vi "Test Worker Waiting After Completing Job.vi"(8 "error in (no error)":errorcluster, 11 "Barista Test in":refnum<class "Barista Test.lvclass">) -> (0 "error out":errorcluster, 3 "Barista Test out":refnum<class "Barista Test.lvclass">)   [LabVIEW 2020, in "Barista Test.lvclass"]
uses:
  Barista Test.lvclass
  C:/Users/anton/Documents/GitHub/Triarc-Examples/Coffee Shop/Worker Test/Worker Test.lvclass
  C:/Program Files (x86)/National Instruments/LabVIEW 2020/vi.lib/Asteme/LUnit/Test Case.lvclass
  Stub Job Processor/Stub Job Handler.lvclass
  C:/Users/anton/Documents/GitHub/Triarc-Examples/Coffee Shop/Process Job/Job Handler.lvclass
  Stub Pick Up Order/Stub Pick Up Order.lvclass
  C:/Users/anton/Documents/GitHub/Triarc-Examples/Coffee Shop/Pick Up Order/Pick Up Order.lvclass
  Support/Beverages/Beverage/Beverage.lvclass
  <vilib>/Asteme/Triarc Framework/Process/Process.lvclass/Process.ctl
  <vilib>/Asteme/LUnit/Test Case.lvclass/Test Case.ctl
  <vilib>/Asteme/LUnit/LUnit Assertion Result.lvclass/LUnit Assertion Result.ctl
  <vilib>/Asteme/Triarc Framework Test Suite/Support/Execution timer.vi
  <vilib>/Asteme/Triarc Framework/Process/Private/SubVIs/Wait for finish.vi
  <vilib>/Asteme/Triarc Framework/Process/Protected/Messaging/Enqueue Message.vi
  <vilib>/Asteme/Triarc Framework/Process/Private/SubVIs/Set Lifecycle State.vi
  <vilib>/Asteme/Triarc Framework/Process/Public/Lifecycle/Get Lifecycle State.vi
  <vilib>/Asteme/LUnit/Palette/Pass If.vi
  <vilib>/Asteme/LUnit/Set Assertion Type.vi
  <vilib>/AdvancedString/1D String Array to Delimited String.vi
  <vilib>/Utility/error.llb/Clear Errors.vi
  <vilib>/Asteme/LUnit/Palette/Fail.vi
  <vilib>/Asteme/LUnit/Palette/Pass.vi
  <vilib>/Asteme/LUnit/LUnit Write Assertion Type.vi
  <vilib>/Asteme/LUnit/Add test result.vi
  <vilib>/Asteme/LUnit/LUnit Write Passed.vi
  <vilib>/Asteme/LUnit/LUnit Get Test Case.vi
  <vilib>/Asteme/LUnit/Assertion Result/LUnit Get Test Name.vi
  <vilib>/Asteme/LUnit/LUnit Write Message.vi
  <vilib>/Asteme/LUnit/LUnit Write Description.vi
  <vilib>/Asteme/LUnit/Read Test Case Name.vi
  Worker/Worker.lvclass
  C:/Program Files (x86)/National Instruments/LabVIEW 2020/vi.lib/Asteme/Triarc Framework/Process/Process.lvclass
  <vilib>/Asteme/Triarc Framework Test Suite/Support/Event Helpers/Dequeue Event Message.vi
  <vilib>/Utility/error.llb/Error Cluster From Error Code.vi
  <vilib>/Asteme/LUnit/LUnit Assertion Result.lvclass
  <vilib>/Asteme/Triarc Framework/Process/Process.lvclass
  Worker Test/Worker Test.lvclass
  <vilib>/Asteme/Triarc Framework Test Suite/Support/Event Helpers/Event Helpers.lvlib
  <vilib>/Asteme/LUnit/Test Case.lvclass
  Support/Order Item/Order Item.lvclass
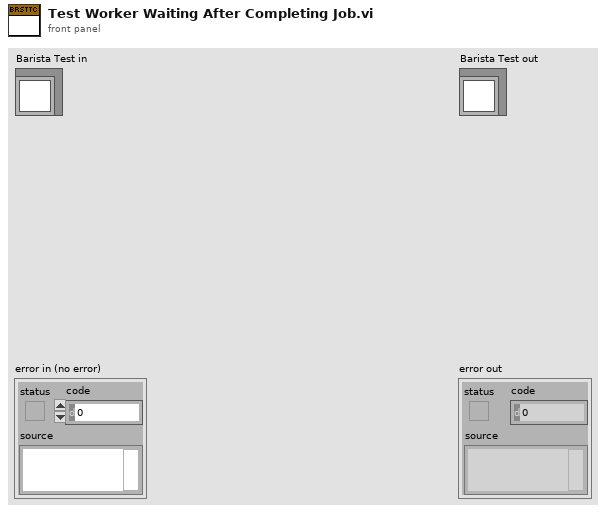
[diagram p1: front panel]
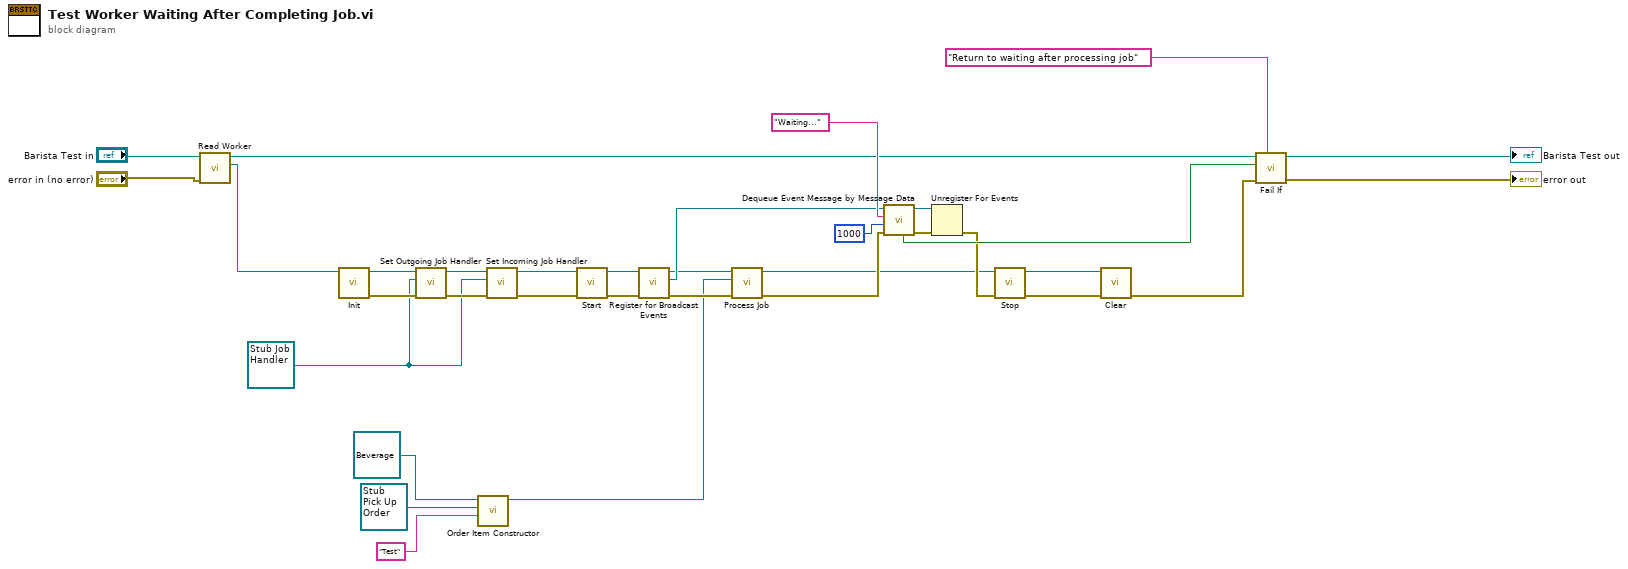
[diagram p0: block diagram]
diagram:
  w1 = refnum<class "Stub Job Handler.lvclass"> refnum ("Stub Job Processor.lvclass")
  n1 = call "Read Worker.vi"("error in (no error)"="error in (no error)", "Worker Test in"="Barista Test in") -> ("Worker"=w7:refnum<class "Worker.lvclass">, "Worker Test out"=w6:refnum<class "Barista Test.lvclass">)  [unwired: 7 in, 1 out]
  n2 = call-dynamic "Init.vi"("View In"=w7) -> ("error out"=w26:errorcluster, "View Out"=w25:refnum<class "Worker.lvclass">)  [unwired: 9 in]
  n3 = call "Set Outgoing Job Handler.vi"("error in (no error)"=w26, "Work Dispatcher"=w1, "Worker In"=w25) -> ("error out"=w30:errorcluster, "Worker Out"=w27:refnum<class "Worker.lvclass">)  [unwired: 7 in]
  n4 = call "Order Item Constructor.vi"("Cust Name"="Test", "Pick Up Order.lvclass"=refnum<class "Stub Pick Up Order.lvclass"> refnum ("Stub Pick Up Order.lvclass"), "Beverage"=refnum<class "Beverage.lvclass"> refnum) -> ("Order Item"=w2:refnum<class "Order Item.lvclass">)  [unwired: 7 in, 1 out]
  n5 = call "Set Incoming Job Handler.vi"("error in (no error)"=w30, "Job Handler"=w1, "Worker In"=w27) -> ("error out"=w29:errorcluster, "Worker Out"=w28:refnum<class "Worker.lvclass">)  [unwired: 7 in]
  n6 = call <vilib>:"Start.vi"("error in (no error)"=w29, "Process In"=w28) -> ("error out"=w10:errorcluster, "Process Out"=w14:refnum<class "Worker.lvclass">)  [unwired: 8 in]
  n7 = call <vilib>:"Register for Broadcast Events.vi"("error in (no error)"=w10, "Process In"=w14) -> ("error out"=w13:errorcluster, "Event Registration Refnum Out"=w18:refnum<event-registration>, "Process Out"=w15:refnum<class "Worker.lvclass">)  [unwired: 7 in]
  n8 = call-dynamic "Process Job.vi"("error in (no error)"=w13, "Job"=w2, "Worker In"=w15) -> ("error out"=w17:errorcluster, "Worker Out"=w16:refnum<class "Worker.lvclass">)  [unwired: 7 in]
  n9 = call <vilib>:"Dequeue Event Message by Message Data.vi"("error in (no error)"=w17, "Timeout (-1)"=1000, "Message Data"="Waiting...", "Event Registration Refnum"=w18) -> ("error out"=w21:errorcluster, "Event Registration Refnum Out"=w23:refnum<event-registration>, "Timed Out?"=w24:bool)  [unwired: 3 in, 2 out]
  n10 = Unregister For Events(event registration refnum=w23, error in=w21) -> (error out=w22:errorcluster)
  n11 = call <vilib>:"Stop.vi"("error in (no error)"=w22, "Process In"=w16) -> ("error out"=w9:errorcluster, "Process Out"=w8:refnum<class "Worker.lvclass">)  [unwired: 7 in, 1 out]
  n12 = call-dynamic "Clear.vi"("error in (no error)"=w9, "View In"=w8) -> ("error out"=w11:errorcluster)  [unwired: 9 in]
  n13 = call <vilib>:"Fail If.vi"("Description"="Return to waiting after processing job", "error in (no error)"=w11, "Fail?"=w24, "Test Case In"=w6) -> ("error out"=→"error out":errorcluster, "Test Case Out"=→"Barista Test out":refnum<class "Barista Test.lvclass">)  [unwired: 6 in]
